vi "get readout test data.vi"(8 "error in (no error)":errorcluster, 11 "path":path=path "C:/Users/dvh-collab-user/Desktop/20230313 Robert sample/tmp.hdf5") -> (0 "error out":errorcluster, 1 "q wave":dbl[][](array[numeric]), 2 "i wave":dbl[][](array[numeric]), 3 "Integral out":dbl[][](array[numeric]))   [LabVIEW 2021]
uses:
  <vilib>/Utility/miscctls.llb/LVRectTypeDef.ctl
  <vilib>/UPVI/lvhdf5/group.llb/H5G_obj_t.ctl
  <vilib>/UPVI/lvhdf5/file.llb/LVH5F Operation.ctl
  <vilib>/UPVI/lvhdf5/dataset.llb/LVH5D Operation.ctl
  <vilib>/UPVI/lvhdf5/identifier.llb/Not an HDF5 Refnum Constant.vi
  <vilib>/UPVI/lvhdf5/file.llb/H5Fopen.vi
  <vilib>/UPVI/lvhdf5/utility.llb/Select HDF5 Dialog.vi
  <vilib>/UPVI/lvhdf5/utility.llb/Select HDF5 Dialog (File and Object).vi
  <vilib>/UPVI/lvhdf5/dataset.llb/Simple H5Dread (Variant).vi
  <vilib>/UPVI/lvhdf5/attribute.llb/Read Multiple Attributes (Variant).vi
  <vilib>/UPVI/lvhdf5/common.llb/To HDF5 Ref.vi
  <vilib>/UPVI/lvhdf5/dataset.llb/H5Dclose.vi
  <vilib>/UPVI/lvhdf5/utility.llb/Select HDF5 Dialog (Object Only).vi
  <vilib>/UPVI/lvhdf5/dataset.llb/Read Dataset and All Attributes.xnode
  <vilib>/UPVI/lvhdf5/library.llb/HDF5 Ref.ctl
  <vilib>/UPVI/lvhdf5/library.llb/HDF5 Ref.lvclass
  <vilib>/UPVI/lvhdf5/dataset.llb/OpenCreateReplace Dataset.vi
  <vilib>/UPVI/lvhdf5/dataset.llb/H5Dget_space.vi
  <vilib>/UPVI/lvhdf5/dataspace.llb/H5Sget_simple_extent_dims.vi
  <vilib>/UPVI/lvhdf5/dataspace.llb/H5Sselect_hyperslab.vi
  <vilib>/UPVI/lvhdf5/dataset.llb/H5Dread (Variant).vi
  <vilib>/UPVI/lvhdf5/attribute.llb/private/LVH5AreadWDTAttrs.vi
  <vilib>/UPVI/lvhdf5/dataspace.llb/H5Sclose.vi
  <vilib>/Utility/error.llb/Error Cluster From Error Code.vi
  <vilib>/Utility/Data Type/Get Type Information.vi
  <vilib>/Utility/Data Type/NI_Data Type.lvlib
  <vilib>/Utility/Data Type/Get Cluster Information.vi
  <vilib>/UPVI/lvhdf5/attribute.llb/Attribute Array to Cluster.xnode
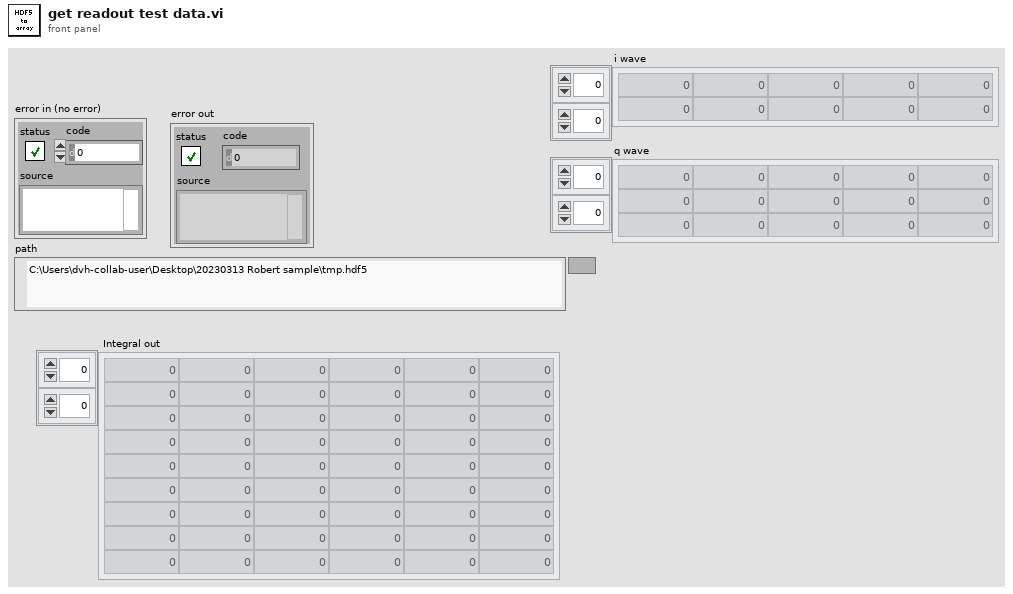
[diagram p1: front panel]
types:
  T1 = typedef "HDF5 Ref.ctl" = refnum<class "HDF5 Ref.lvclass">
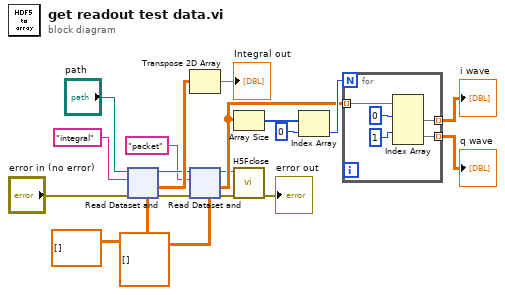
[diagram p0: block diagram]
diagram:
  n1 = xnode "Read Dataset and"("Dataset Path"="integral", "error in (no error)"="error in (no error)", "HDF5 Path or Ref"="path", "Data"=dbl[][] []) -> ("HDF5 Ref out"=w11:T1, "error out"=w12:errorcluster, "Data out"=w14:dbl[][])  [unwired: 2 in, 3 out]
  n2 = Transpose 2D Array(2D array=w14) -> (transposed array=→"Integral out":dbl[][])
  n3 = xnode "Read Dataset and"("Dataset Path"="packet", "error in (no error)"=w12, "HDF5 Path or Ref"=w11, "Data"=dbl[][][] []) -> ("HDF5 Ref out"=w3:T1, "error out"=w2:errorcluster, "Data out"=w5:dbl[][][])  [unwired: 2 in, 3 out]
  n4 = Array Size(array=w5) -> (size(s)=w8:i32[])
  n5 = call <vilib>:"H5Fclose.vi"("error in (no error)"=w2, "HDF5 Ref"=w3) -> ("error out"=→"error out":errorcluster)  [unwired: 7 in]
  n6 = Index Array(array=w8, index=0) -> (element=w6:i32)
  n7 = for {
    N: w6 -> [_]
    tunnel: w5 -> [w24] mode=indexing
    tunnel: [w21] -> w1 mode=indexing
    tunnel: [w20] -> w4 mode=indexing
    n8 = Index Array(array=w24, index (row) #1=0 ("index (row)"), index (row) #2=1 ("index (row)")) -> (element #1=w21:dbl[], element #2=w20:dbl[])  [unwired: 2 in]
  }
  "i wave" <- w1
  "q wave" <- w4
